vi "ResetRef.vi"(8 "error in (no error)":errorcluster, 10 "Boolean in":refnum<vi>) -> (0 "error out":errorcluster, 2 "Boolean out":refnum<vi>)   [LabVIEW 2017, in "TagDB RefManager.lvlib"]
uses:
  TagDB RefManager.lvlib
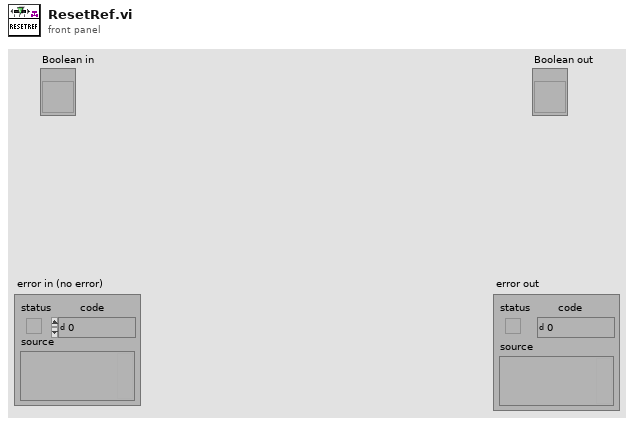
[diagram p1: front panel]
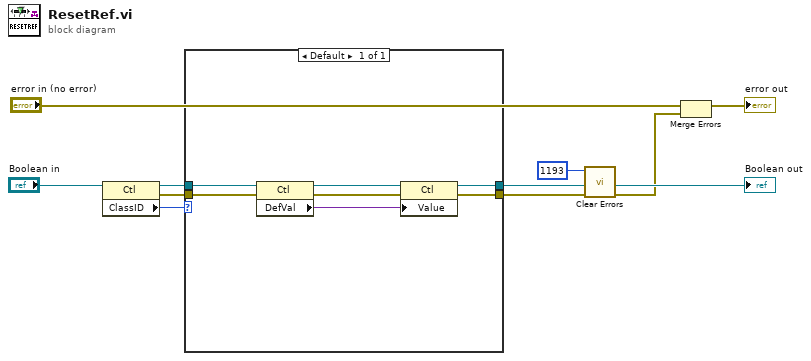
[diagram p0: block diagram]
diagram:
  n1 = property class="Ctl"(reference="Boolean in") -> (reference out=w3:refnum<vi>, error out=w1:errorcluster, "ClassID"=w2:u32)  [unwired: 1 in]
  n2 = case shown="Default" w2 {
    tunnel: [w14] -> w7
    tunnel: [w13] -> w6
    tunnel: w3 -> [w12]
    tunnel: w1 -> [w11]
    frame Default {
      n3 = property class="Ctl"(reference=w12, error in=w11) -> (reference out=w17:refnum<vi>, error out=w15:errorcluster, "DefVal"=w16:variant)
      n4 = property class="Ctl"(reference=w17, error in=w15, "Value"=w16) -> (reference out=w13:refnum<vi>, error out=w14:errorcluster)
    }
  }
  "Boolean out" <- w6
  n5 = call <vilib>:"Clear Errors.vi"("error in (no error)"=w7, "specific error code to clear (0: all)"=1193) -> ("error out"=w5:errorcluster)  [unwired: 4 in, 1 out]
  n6 = Merge Errors("error in (no error)", w5) -> (→"error out":errorcluster)
